vi "getConstants.vi"(0 "AnalogOutput in":refnum<class "AnalogOutput.lvclass">, 1 "error in (no error)":errorcluster) -> (2 "AnalogOutput out":refnum<class "AnalogOutput.lvclass">, 3 "Constants":T1, 4 "error out":errorcluster)   [LabVIEW 2011, in "Hardware.lvlib" / "Channels.lvlib" / "AnalogOutput.lvclass"]
doc: "Returns the Constants value.\n\nConfiguration Type (Differential, Pseudodifferential, RSE)\nOutput Type (Voltage, Current, Standard Function (Sine, Square, Triangle))"
uses:
  AnalogOutput.lvclass
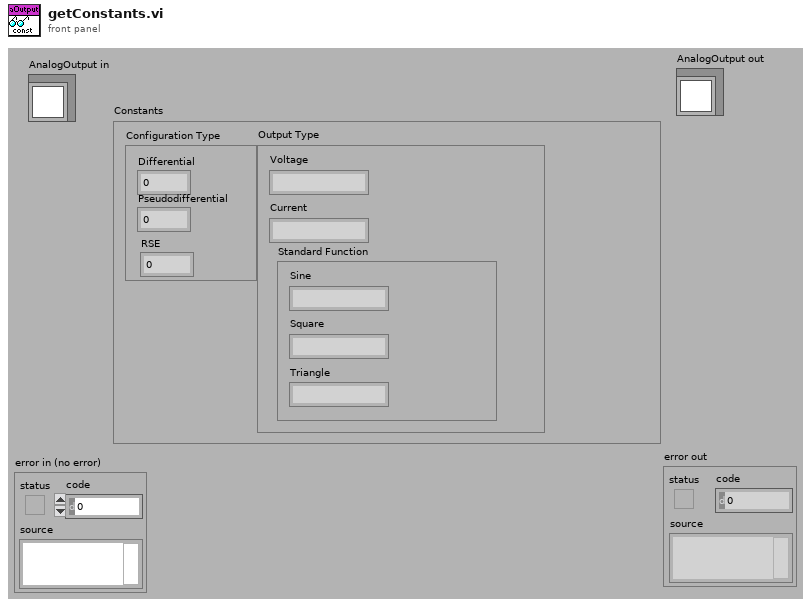
[diagram p1: front panel]
types:
  T1 = cluster{"Configuration Type":cluster{"Differential":i16, "Pseudodifferential":i16, "RSE":dbl}, "Output Type":cluster{"Voltage":string, "Current":string, "Standard Function ":cluster{"Sine":string, "Square":string, "Triangle":string}}}
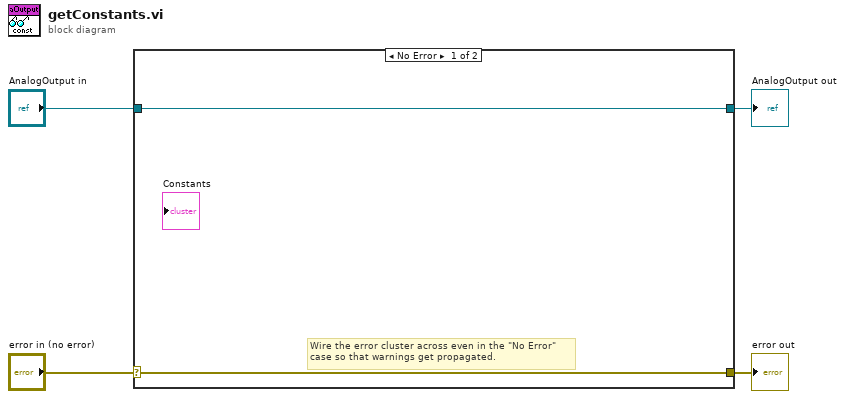
[diagram p0: block diagram]
diagram:
  n1 = case shown="No Error" "error in (no error)" {
    selector: "error in (no error)" -> [w5 w8]
    tunnel: [w5 w8] -> w3
    tunnel: [w6 w7] -> w1
    tunnel: "AnalogOutput in" -> [w6 w7]
    frame No Error {
      # "Wire the error cluster across even in the \"No Error\"\ncase so that warnings get propagated."
    }
    frame Error {
    }
  }
  "error out" <- w3
  "AnalogOutput out" <- w1
